vi "reg.vi"(1 "C":bool, 2 "WRITE":bool, 3 "INPUT":T2, 4 "R":bool) -> (0 "OUTPUT":T1)   [LabVIEW 2013]
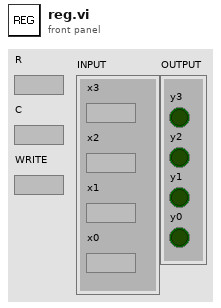
[diagram p1: front panel]
types:
  T1 = cluster{"y3":bool, "y2":bool, "y1":bool, "y0":bool}
  T2 = cluster{"x3":bool, "x2":bool, "x1":bool, "x0":bool}
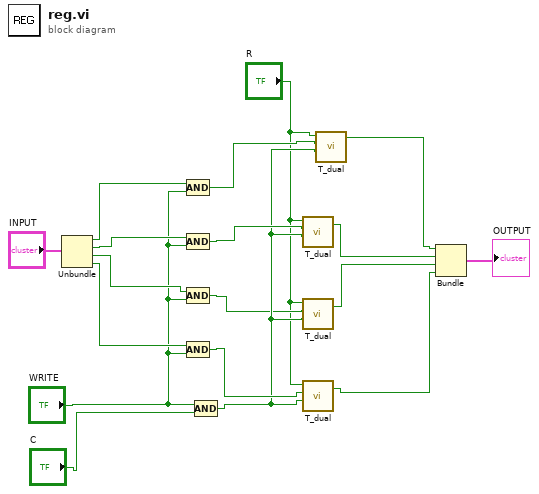
[diagram p0: block diagram]
diagram:
  n1 = Unbundle("INPUT") -> ("x3"=w17:bool, "x2"=w16:bool, "x1"=w15:bool, "x0"=w14:bool)
  n2 = Compound Arithmetic op=AND(w17, "WRITE") -> (w9:bool)
  n3 = Compound Arithmetic op=AND(w16, "WRITE") -> (w8:bool)
  n4 = Compound Arithmetic op=AND(w15, "WRITE") -> (w2:bool)
  n5 = Compound Arithmetic op=AND(w14, "WRITE") -> (w4:bool)
  n6 = Compound Arithmetic op=AND("WRITE", "C") -> (w3:bool)
  n7 = call "T_dual.vi"("C"=w3, "D"=w8, "R"="R") -> ("Q"=w7:bool)  [unwired: 1 in, 1 out]
  n8 = call "T_dual.vi"("C"=w3, "D"=w2, "R"="R") -> ("Q"=w6:bool)  [unwired: 1 in, 1 out]
  n9 = call "T_dual.vi"("C"=w3, "D"=w4, "R"="R") -> ("Q"=w5:bool)  [unwired: 1 in, 1 out]
  n10 = call "T_dual.vi"("C"=w3, "D"=w9, "R"="R") -> ("Q"=w10:bool)  [unwired: 1 in, 1 out]
  n11 = Bundle("Q"=w10, "Q"=w7, "Q"=w6, "Q"=w5) -> (→"OUTPUT":cluster{"Q":bool, "Q":bool, "Q":bool, "Q":bool})  [unwired: 1 in]
